vi "construct.vi"(8 "error in (no error)":errorcluster, 9 "configuration name":string, 10 "load config file?":bool=TRUE, 11 "DL090202ScanHead in":refnum<class "ScanHeadDL090202.lvclass">) -> (0 "error out":errorcluster, 3 "DL090202ScanHead out":refnum<class "ScanHeadDL090202.lvclass">)   [LabVIEW 2010, in "ScanHeadDL090202.lvclass"]
uses:
  ScanHeadDL090202.lvclass
  Clock/GenericClock/GenericClock/GenericClock.lvclass
  SignalWriter/GenericSignalWriter/GenericSignalWriter/GenericSignalWriter.lvclass
  common/classes/GenericComponent/GenericComponent/GenericComponent.lvclass
  common/classes/ErrorController/ErrorController/ErrorController.lvclass
  GenericScanHead/GenericScanHead/GenericScanHead.lvclass
  DigitalOut/GenericDigitalOut/GenericDigitalOut/GenericDigitalOut.lvclass
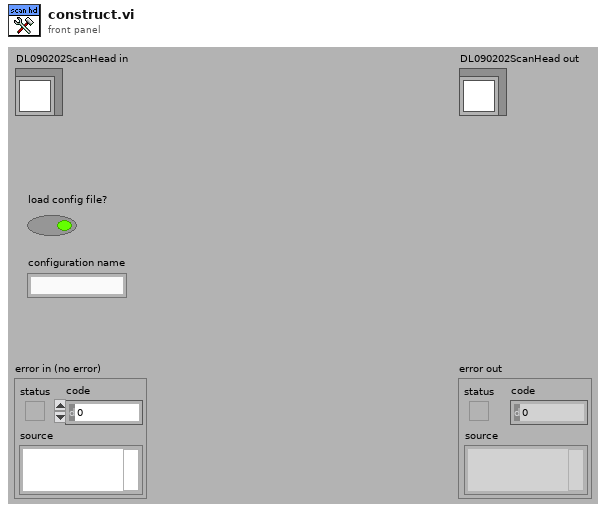
[diagram p1: front panel]
types:
  T1 = typedef "plugin_specification.ctl" = cluster{"class path":string, "configuration":string, "label":string, "settings name":string}
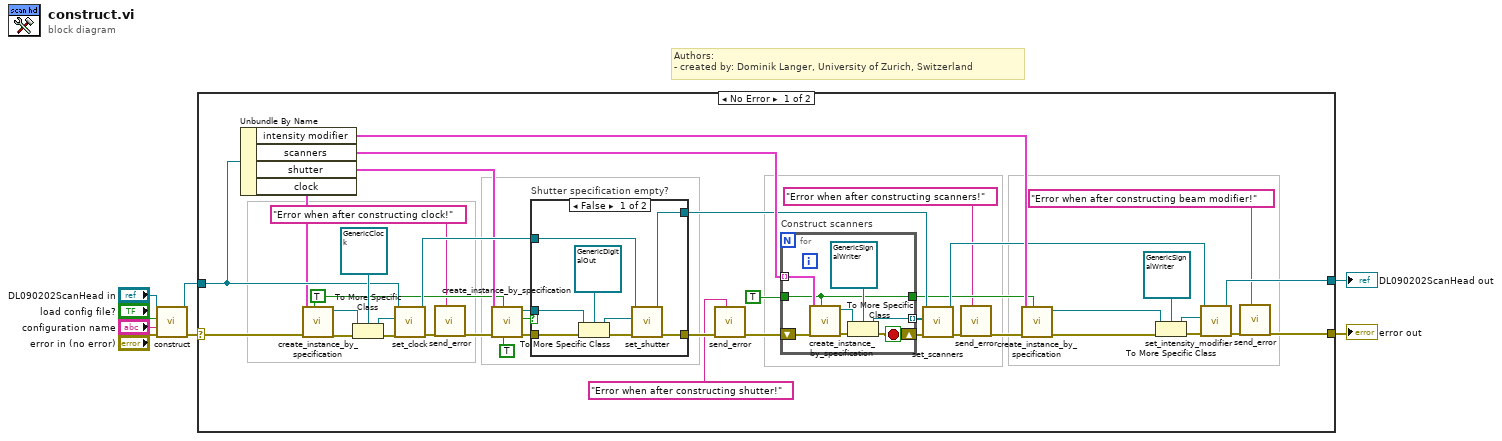
[diagram p0: block diagram]
diagram:
  # "Authors: \n- created by: Dominik Langer, University of Zurich, Switzerland"
  n1 = call-parent "construct.vi"("error in (no error)"="error in (no error)", "configuration name"="configuration name", "load config file?"="load config file?", "GenericPlugin in"="DL090202ScanHead in") -> ("error out"=w4:errorcluster, "GenericPlugin out"=w3:refnum<class "ScanHeadDL090202.lvclass">)  [unwired: 6 out]
  n2 = case shown="No Error" w4 {
    selector: w4 -> [w37 w68]
    tunnel: w3 -> [w46 w69]
    tunnel: [w14 w68] -> w2
    tunnel: [w38 w69] -> w1
    frame No Error {
      w28 = TRUE ("call constructor?")
      n3 = Unbundle By Name(w46) -> ("intensity modifier"=w47:T1, "scanners"=w48:T1[], "shutter"=w31:T1, "clock"=w34:T1)
      n4 = call "create_instance_by_specification.vi"("call constructor?"=w28, "error in (no error)"=w37, "component specification"=w34) -> ("error out"=w36:errorcluster, "GenericPlugin out"=w35:refnum<class "GenericComponent.lvclass">)  [unwired: 6 in, 1 out]
      n5 = To More Specific Class(target class=refnum<class "GenericClock.lvclass"> refnum ("GenericClock.lvclass"), reference=w35, error in=w36) -> (specific class reference=w32:refnum<class "GenericClock.lvclass">, error out=w33:errorcluster)
      n6 = call-dynamic "set_clock.vi"("error in (no error)"=w33, "GenericClock.lvclass"=w32, "DL090202ScanHead.lvclass in"=w46) -> ("error out"=w23:errorcluster, "DL090202ScanHead.lvclass out"=w45:refnum<class "ScanHeadDL090202.lvclass">)  [unwired: 7 out]
      n7 = call "send_error.vi"("additional message"="Error when after constructing clock!", "error in (no error)"=w23) -> ("error out"=w22:errorcluster)  [unwired: 9 in]
      n8 = call "create_instance_by_specification.vi"("be tolerant against empty specification?"=TRUE, "call constructor?"=w28, "error in (no error)"=w22, "component specification"=w31) -> ("error out"=w30:errorcluster, "empty specification!"=w10:bool, "GenericPlugin out"=w29:refnum<class "GenericComponent.lvclass">)  [unwired: 5 in]
      n9 = case "Shutter specification empty?" shown="False" w10 {
        tunnel: w45 -> [w57 w59]
        tunnel: [w56 w59] -> w42
        tunnel: w30 -> [w55 w58]
        tunnel: w29 -> [w53 _]
        tunnel: [w52 w58] -> w20
        frame False {
          n10 = To More Specific Class(target class=refnum<class "GenericDigitalOut.lvclass"> refnum ("GenericDigitalOut.lvclass"), reference=w53, error in=w55) -> (specific class reference=w50:refnum<class "GenericDigitalOut.lvclass">, error out=w54:errorcluster)
          n11 = call-dynamic "set_shutter.vi"("error in (no error)"=w54, "GenericDigitalOut.lvclass"=w50, "DL090202ScanHead.lvclass in"=w57) -> ("error out"=w52:errorcluster, "DL090202ScanHead.lvclass out"=w56:refnum<class "ScanHeadDL090202.lvclass">)  [unwired: 7 out]
        }
        frame True {
        }
      }
      n12 = call "send_error.vi"("additional message"="Error when after constructing shutter!", "error in (no error)"=w20) -> ("error out"=w19:errorcluster)  [unwired: 9 in]
      n13 = for "Construct scanners" {
        shift-right: [w60] -> w44
        shift-left: w19 -> [w66]
        tunnel: w48 -> [w62] mode=indexing
        tunnel: [w63] -> w43 mode=indexing
        tunnel: TRUE ("call constructor?") -> [w61]
        tunnel: [w61] -> w27
        stop <- w60 stop-if-true
        n14 = call "create_instance_by_specification.vi"("call constructor?"=w61, "error in (no error)"=w66, "component specification"=w62) -> ("error out"=w64:errorcluster, "GenericPlugin out"=w65:refnum<class "GenericComponent.lvclass">)  [unwired: 6 in, 1 out]
        n15 = To More Specific Class(target class=refnum<class "GenericSignalWriter.lvclass"> refnum ("GenericSignalWriter.lvclass"), reference=w65, error in=w64) -> (specific class reference=w63:refnum<class "GenericSignalWriter.lvclass">, error out=w60:errorcluster)
      }
      n16 = call-dynamic "set_scanners.vi"("error in (no error)"=w44, "scanners"=w43, "DL090202ScanHead.lvclass in"=w42) -> ("error out"=w18:errorcluster, "DL090202ScanHead.lvclass out"=w39:refnum<class "ScanHeadDL090202.lvclass">)  [unwired: 7 out]
      n17 = call "send_error.vi"("additional message"="Error when after constructing scanners!", "error in (no error)"=w18) -> ("error out"=w17:errorcluster)  [unwired: 9 in]
      n18 = call "create_instance_by_specification.vi"("call constructor?"=w27, "error in (no error)"=w17, "component specification"=w47) -> ("error out"=w24:errorcluster, "GenericPlugin out"=w25:refnum<class "GenericComponent.lvclass">)  [unwired: 6 in, 1 out]
      n19 = To More Specific Class(target class=refnum<class "GenericSignalWriter.lvclass"> refnum ("GenericSignalWriter.lvclass"), reference=w25, error in=w24) -> (specific class reference=w40:refnum<class "GenericSignalWriter.lvclass">, error out=w41:errorcluster)
      n20 = call-dynamic "set_intensity_modifier.vi"("error in (no error)"=w41, "write signals"=w40, "DL090202ScanHead.lvclass in"=w39) -> ("error out"=w15:errorcluster, "DL090202ScanHead.lvclass out"=w38:refnum<class "ScanHeadDL090202.lvclass">)  [unwired: 7 out]
      n21 = call "send_error.vi"("additional message"="Error when after constructing beam modifier!", "error in (no error)"=w15) -> ("error out"=w14:errorcluster)  [unwired: 9 in]
    }
    frame Error {
    }
  }
  "error out" <- w2
  "DL090202ScanHead out" <- w1
